vi "SetCanUserResize.vi"(0 "reference in":refnum<class "DataGridView.lvclass">, 5 "AllowUserToResizeRows":bool, 7 "AllowUserToResizeColumns":bool, 11 "error in (no error)":errorcluster) -> (4 "reference out":refnum<class "DataGridView.lvclass">, 15 "error out":errorcluster)   [LabVIEW 2018, in "DataGridView.lvclass"]
doc: "Sets the value indicating whether users can resize columns and rows."
uses:
  DataGridView.lvclass
  System.Windows.Forms
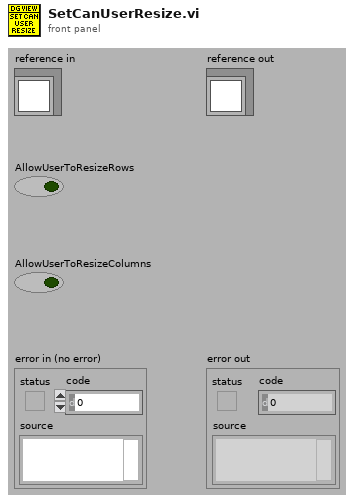
[diagram p1: front panel]
types:
  T1 = typedef "DataGridView.lvclass/ObjectAttributes.ctl" = cluster{"DataGridView":refnum<k24>, "SelectionChangedEvent":refnum<user-event>, "SelectionChanged callback ref":refnum<k27>, "LastSelectedRowIndex":i32}
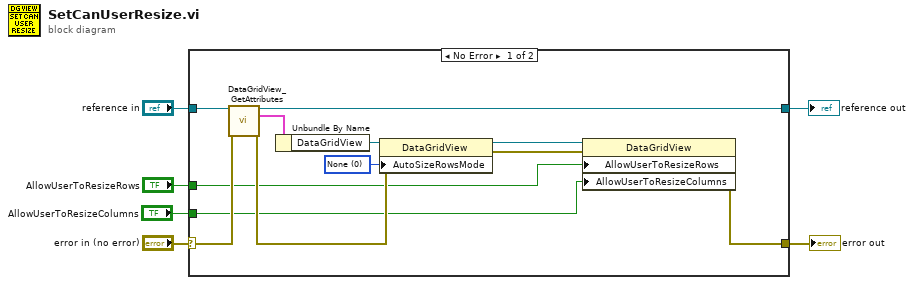
[diagram p0: block diagram]
diagram:
  n1 = case shown="No Error" "error in (no error)" {
    selector: "error in (no error)" -> [w18 w20]
    tunnel: [w9 w20] -> w5
    tunnel: [w15 w19] -> w3
    tunnel: "reference in" -> [w16 w19]
    tunnel: "AllowUserToResizeRows" -> [w8 _]
    tunnel: "AllowUserToResizeColumns" -> [w7 _]
    frame No Error {
      w13 = 0 items=["None"=0, "AllHeaders"=5, "AllCellsExceptHeaders"=6, "AllCells"=7, "DisplayedHeaders"=9, "DisplayedCellsExceptHeaders"=10, "DisplayedCells"=11] ("AutoSizeRowsMode")
      n2 = call "DataGridView_GetAttributes.vi"("reference in"=w16, "error in (no error)"=w18) -> ("reference out"=w15:refnum<class "DataGridView.lvclass">, "Data"=w17:T1, "error out"=w10:errorcluster)  [unwired: 10 in, 1 out]
      n3 = Unbundle By Name(w17) -> ("DataGridView"=w14:refnum<k24>)
      n4 = property class="DataGridView"(reference=w14, error in=w10, "AutoSizeRowsMode"=w13) -> (reference out=w12:refnum<k24>, error out=w11:errorcluster)
      n5 = property class="DataGridView"(reference=w12, error in=w11, "AllowUserToResizeRows"=w8, "AllowUserToResizeColumns"=w7) -> (error out=w9:errorcluster)  [unwired: 1 out]
    }
    frame Error {
    }
  }
  "error out" <- w5
  "reference out" <- w3
